vi "check_boc_rms_freq_char.vi"(7 "Attenuator(dB)":T1, 8 "error in (no error)":errorcluster, 9 "Amplitude (1.0 Vpp)":dbl=1.0 format="%#.4f", 10 "freq":dbl[](array[numeric]), 11 "app_data in":T2) -> (0 "error out":errorcluster, 1 "meas":dbl[][](array[numeric]), 2 "boc_data":sgl[][](array[numeric]), 3 "app_data_out":T2)   [LabVIEW 2017]
uses:
  controls/app_data.ctl
  controls/instruments.ctl
  Unicorn Labview Library/Control/unicorn_Param.ctl
  Unicorn Labview Library/Control/unicorn_conn.ctl
  Unicorn Labview Library/Control/unicorn_JSON.ctl
  Unicorn Labview Library/Control/unicorn_ParamInt.ctl
  Unicorn Labview Library/Control/unicorn_Telemetry.ctl
  Unicorn Labview Library/Control/unicorn_Table.ctl
  Unicorn Labview Library/Control/unicorn_ParamFloat.ctl
  controls/attenuator_dB.ctl
  Unicorn Labview Library/Unicorn Library.lvlib
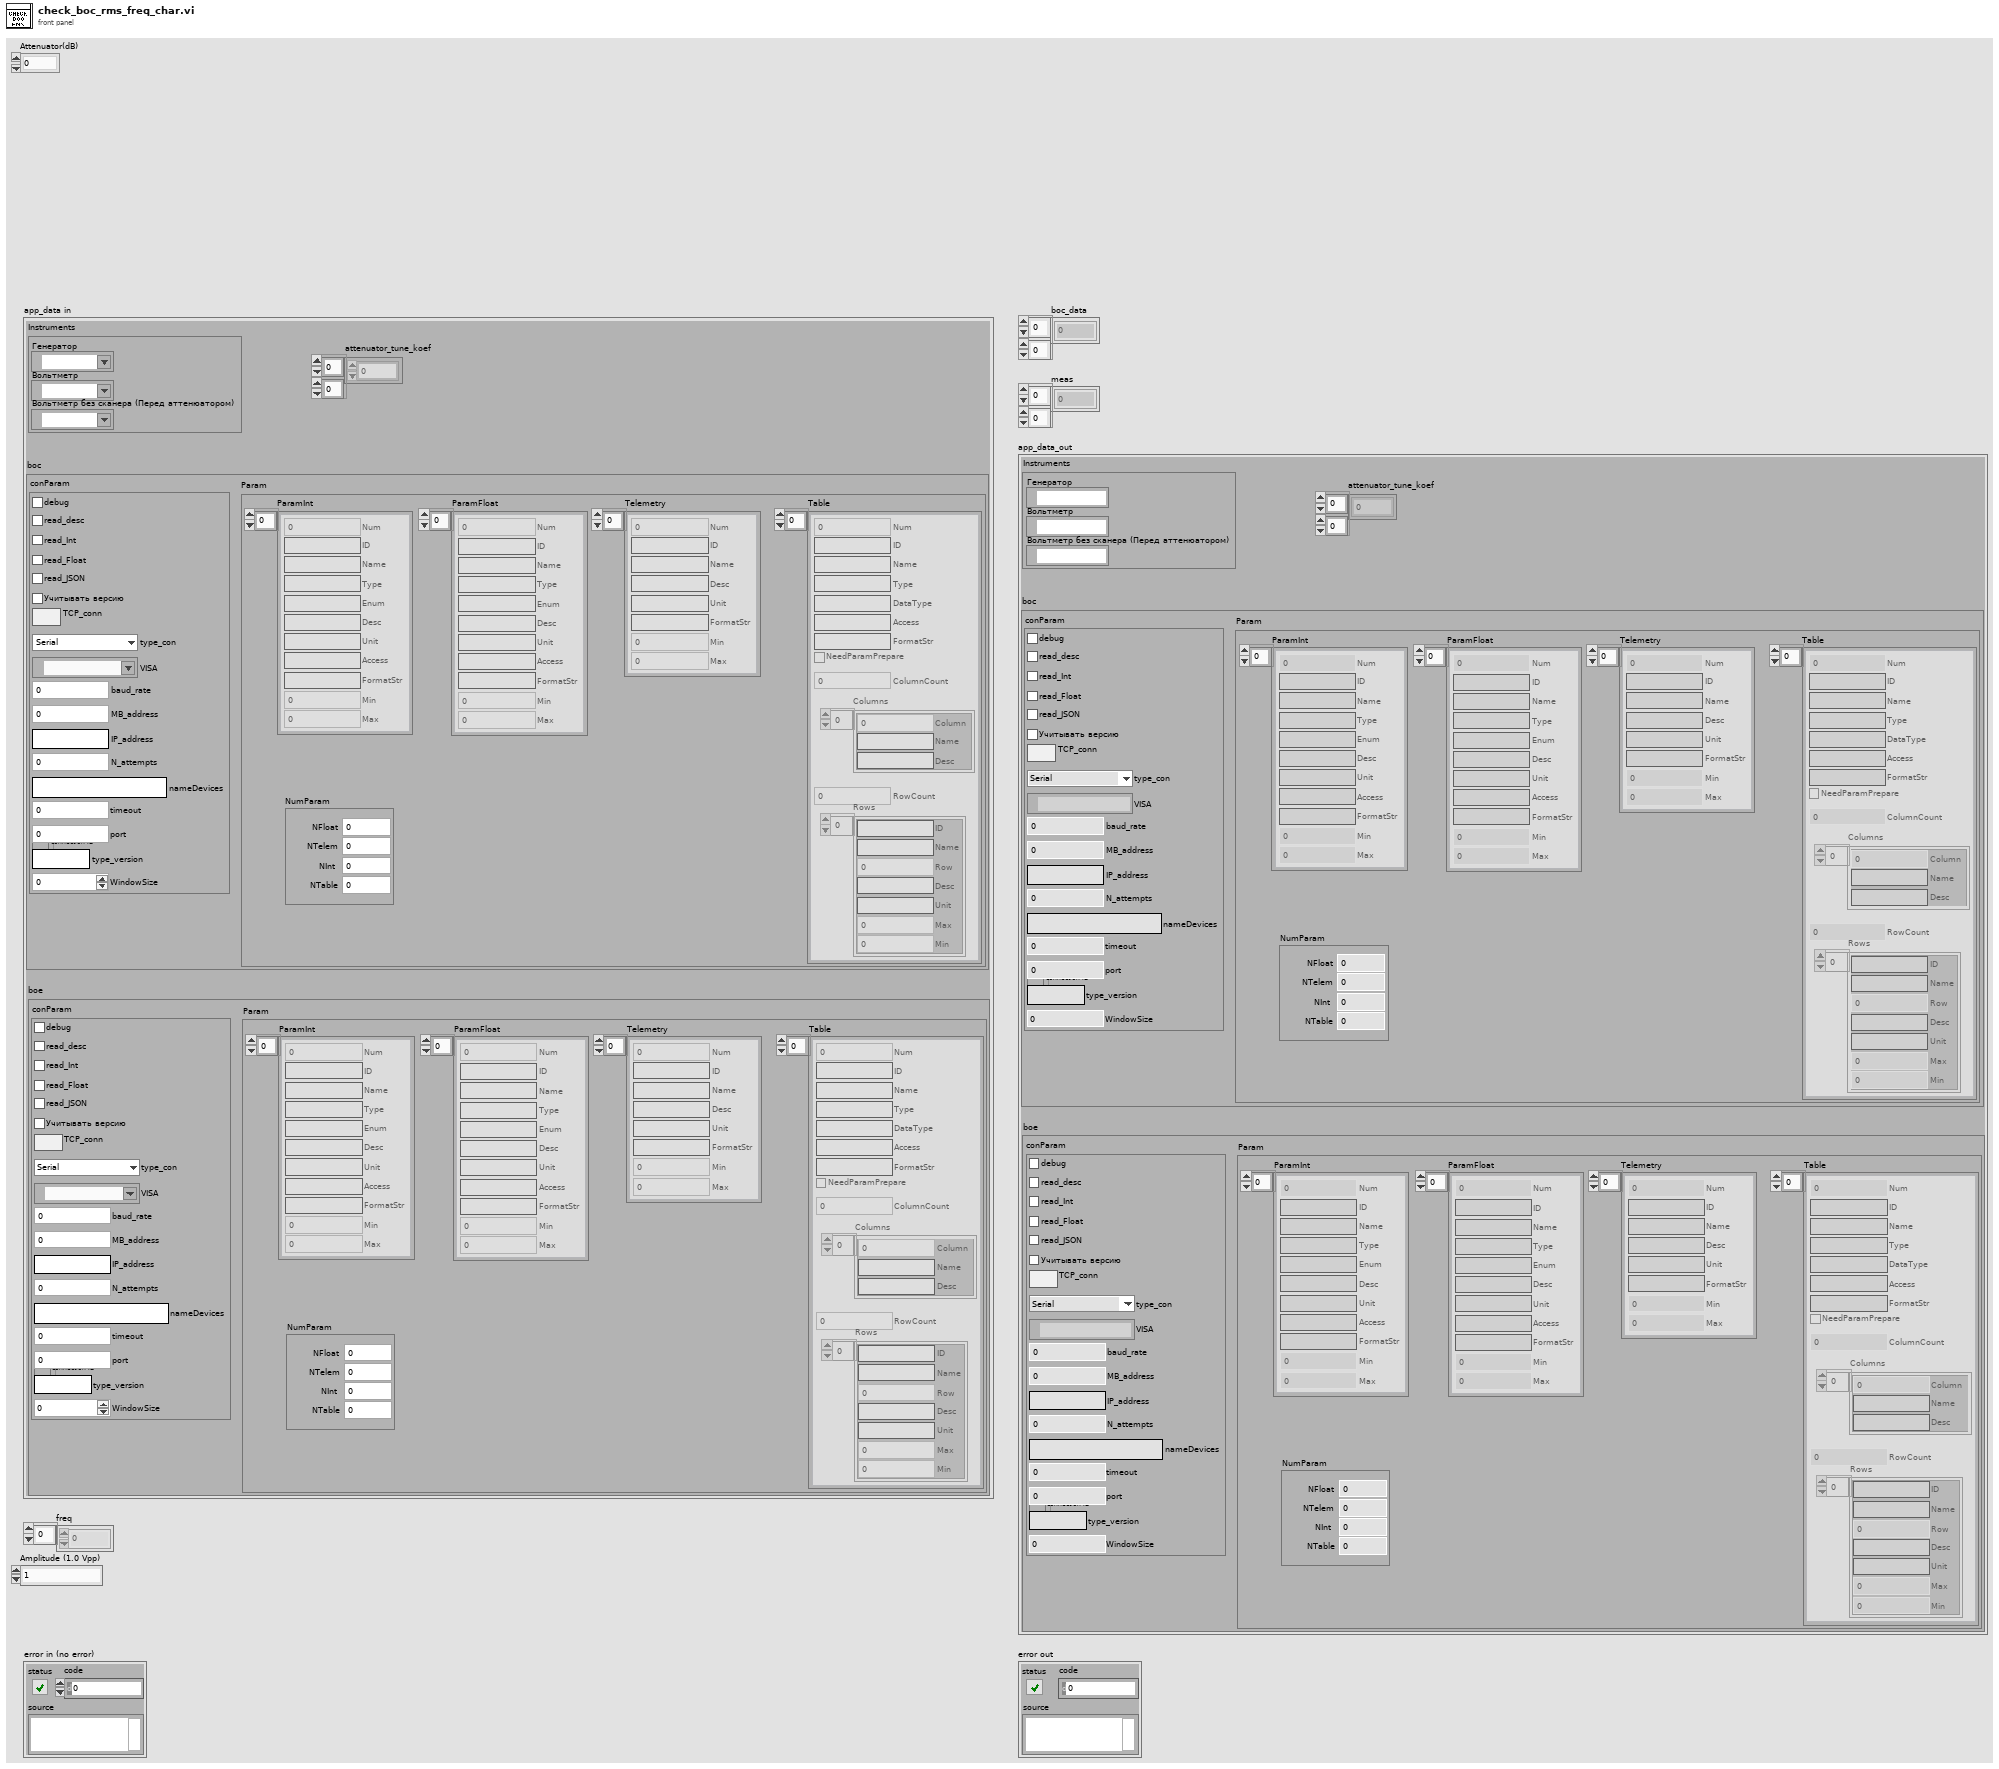
[diagram p1: front panel]
types:
  T1 = typedef "attenuator_dB.ctl" = enum16{"0", "20", "40", "60"}
  T2 = typedef "app_data.ctl" = cluster{"Instruments":T3, "boc":T4, "boe":T4, "attenuator_tune_koef":dbl[][]}
  T3 = typedef "instruments.ctl" = cluster{"generator":refnum<visa-resource-name>, "voltment_with_scaner":refnum<visa-resource-name>, "voltment_without_scaner":refnum<visa-resource-name>}
  T4 = typedef "Unicorn Library.lvlib/unicorn_Param.ctl" = cluster{"conParam":T5, "Param":T6}
  T5 = typedef "Unicorn Library.lvlib/unicorn_conn.ctl" = cluster{"ReadIntParam":bool, "ReadDescrParam":bool, "ReadFloatParam":bool, "debug":bool, "ReadJSON":bool, "IP_address":string, "N_attempts":i32, "type_con":enum16{"Serial", "TCP"}, "MB_address":i32, "VISA":refnum<visa-resource-name>, "connection ID":refnum<k5>, "nameDevices":string, "timeout":i32, "port":u16, "type_version":string, "baud_rate":u32, "VersionControl":bool, "TCP_conn":bool, "WindowSize":i32}
  T6 = typedef "Unicorn Library.lvlib/unicorn_JSON.ctl" = cluster{"NumParam":cluster{"NTelem":i32, "NInt":i32, "NFloat":i32, "NTable":i32}, "ParamInt":T7, "Telemetry":T8, "Table":T9, "ParamFloat":T10}
  T7 = typedef "Unicorn Library.lvlib/unicorn_ParamInt.ctl" = cluster{"ID":string, "Num":i32, "Name":string, "Type":string, "Enum":string, "Desc":string, "Unit":string, "Access":string, "FormatStr":string, "Min":i32, "Max":i32}[]
  T8 = typedef "Unicorn Library.lvlib/unicorn_Telemetry.ctl" = cluster{"ID":string, "Num":i32, "Name":string, "Desc":string, "Unit":string, "FormatStr":string, "Min":i32, "Max":i32}[]
  T9 = typedef "Unicorn Library.lvlib/unicorn_Table.ctl" = cluster{"Num":i32, "Access":string, "ColumnCount":i32, "NeedParamPrepare":bool, "Columns":cluster{"Column":i32, "Desc":string, "Name":string}[], "DataType":string, "FormatStr":string, "ID":string, "Name":string, "RowCount":i32, "Rows":cluster{"Desc":string, "ID":string, "Max":i32, "Min":i32, "Name":string, "Row":i32, "Unit":string}[], "Type":string}[]
  T10 = typedef "Unicorn Library.lvlib/unicorn_ParamFloat.ctl" = cluster{"ID":string, "Num":i32, "Name":string, "Type":string, "Enum":string, "Desc":string, "Unit":string, "Access":string, "FormatStr":string, "Min":i32, "Max":i32}[]
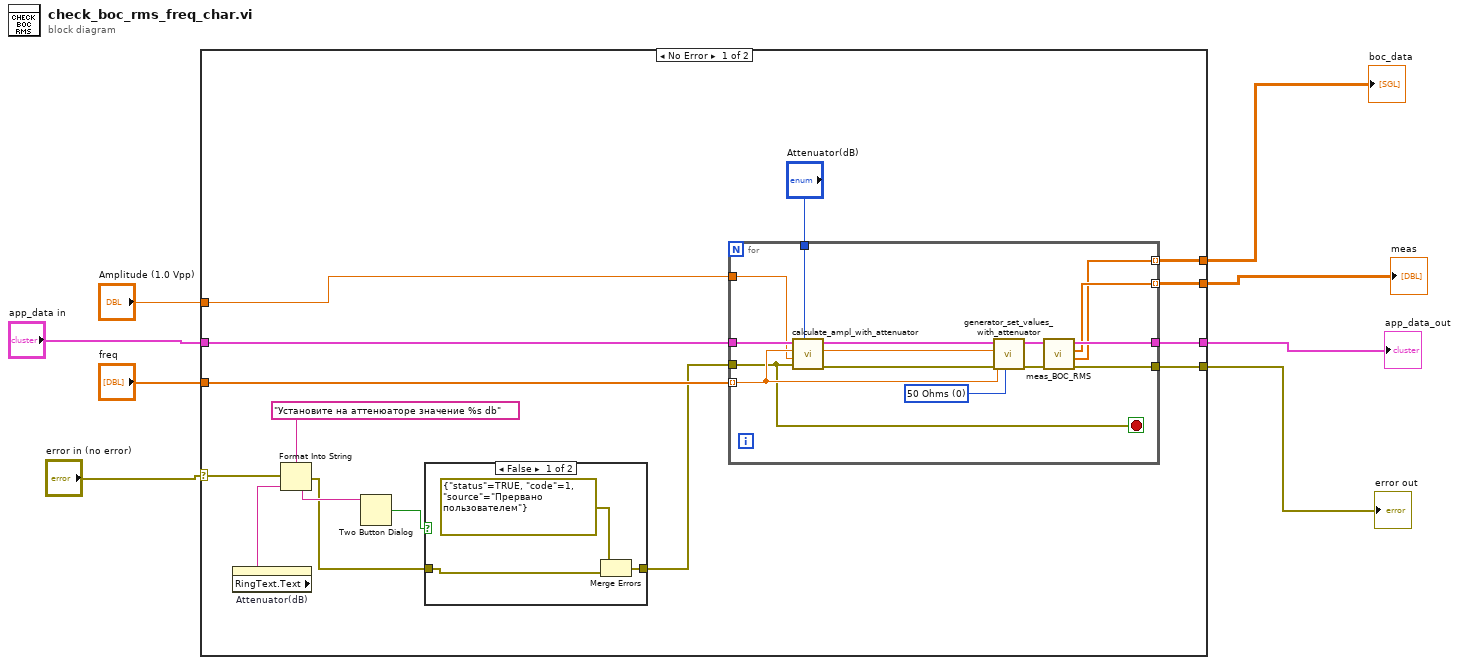
[diagram p0: block diagram]
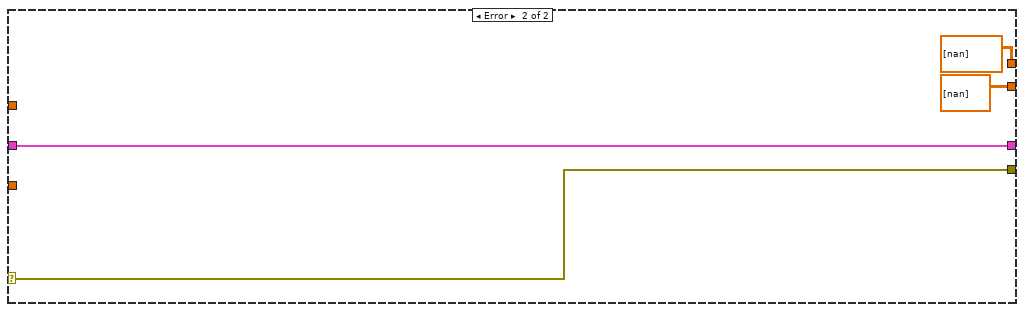
[diagram p3: hidden frame]
diagram:
  n1 = case shown="No Error" "error in (no error)" {
    selector: "error in (no error)" -> [w9 w46]
    tunnel: "freq" -> [w23 _]
    tunnel: [w22 dbl[][] [[nan]] ("meas")] -> w7
    tunnel: [w21 sgl[][] [[nan]] ("boc_data")] -> w6
    tunnel: [w20 w46] -> w5
    tunnel: [w19 w45] -> w4
    tunnel: "Amplitude (1.0 Vpp)" -> [w18 _]
    tunnel: "app_data in" -> [w17 w45]
    frame No Error {
      n2 = property on="Attenuator(dB)" class="Enum (strict)"() -> ("RingText.Text"=w15:string)  [unwired: 2 in, 2 out]
      n3 = Format Into String(format string="Установите на аттенюаторе значение %s db", error in=w9, w15) -> (resulting string=w14:string, error out=w11:errorcluster)  [unwired: 1 in]
      n4 = Two Button Dialog(message=w14) -> (T button?=w13:bool)  [unwired: 2 in]
      n5 = case shown="False" w13 {
        tunnel: w11 -> [w24 w27]
        tunnel: [w26 w27] -> w10
        frame False {
          n6 = Merge Errors(errorcluster {"status"=TRUE, "code"=1, "source"="Прервано пользователем"} ("error constant"), w24) -> (w26:errorcluster)
        }
        frame True {
        }
      }
      n7 = for {
        tunnel: w23 -> [w35] mode=indexing
        tunnel: [w38] -> w22 mode=indexing
        tunnel: [w37] -> w21 mode=indexing
        tunnel: w10 -> [w33]
        tunnel: [w39] -> w20
        tunnel: w17 -> [w36]
        tunnel: [w40] -> w19
        tunnel: w18 -> [w30]
        tunnel: "Attenuator(dB)" -> [w29]
        stop <- w33 stop-if-true
        w28 = u16 0 items=["50 Ohms", "High Impedance"] ("Impedance (0: 50 Ohms)")
        n8 = call "calculate_ampl_with_attenuator.vi"("Attenuator(dB)"=w29, "error in"=w33, "Amplitude_in"=w30, "frequency"=w35, "app_data in in"=w36) -> ("error out"=w34:errorcluster, "Amplitude_out"=w32:dbl, "app_data out"=w31:T2)  [unwired: 4 in]
        n9 = call "generator_set_values_with_attenuator.vi"("Impedance (0: 50 Ohms)"=w28, "error in (no error)"=w34, "Frequency (1000 Hz)"=w35, "Amplitude (1.0 Vpp)"=w32, "app_data"=w31) -> ("error out"=w41:errorcluster, "output cluster"=w42:T2)  [unwired: 5 in]
        n10 = call "meas_BOC_RMS.vi"("error in (no error)"=w41, "output cluster in"=w42) -> ("error out"=w39:errorcluster, "boc_data"=w37:sgl[], "meas"=w38:dbl[], "output cluster out"=w40:T2)  [unwired: 6 in]
      }
    }
    frame Error {
    }
  }
  "meas" <- w7
  "boc_data" <- w6
  "error out" <- w5
  "app_data_out" <- w4
